vi "Test Person Broadcasts Status on Start.vi"(8 "error in (no error)":errorcluster, 11 "Person Test In":refnum<class "Person Test.lvclass">) -> (0 "error out":errorcluster, 3 "Person Test Out":refnum<class "Person Test.lvclass">)   [LabVIEW 2020, in "Person Test.lvclass"]
uses:
  Person Test/Person Test.lvclass
  C:/Program Files (x86)/National Instruments/LabVIEW 2020/vi.lib/Asteme/LUnit/Test Case.lvclass
  Processes/People/Person/Person.lvclass
  C:/Program Files (x86)/National Instruments/LabVIEW 2020/vi.lib/Asteme/Triarc Framework/Process/Process.lvclass
  <vilib>/Asteme/Triarc Framework/Process/Process.lvclass/Process.ctl
  <vilib>/Asteme/LUnit/Test Case.lvclass/Test Case.ctl
  <vilib>/Asteme/LUnit/LUnit Assertion Result.lvclass/LUnit Assertion Result.ctl
  <vilib>/Asteme/Triarc Framework Test Suite/Support/Execution timer.vi
  <vilib>/Asteme/Triarc Framework/Process/Private/SubVIs/Wait for finish.vi
  <vilib>/Asteme/Triarc Framework/Process/Protected/Messaging/Enqueue Message.vi
  <vilib>/Asteme/Triarc Framework/Process/Private/SubVIs/Set Lifecycle State.vi
  <vilib>/Asteme/Triarc Framework/Process/Public/Lifecycle/Get Lifecycle State.vi
  <vilib>/Asteme/LUnit/Palette/Fail.vi
  <vilib>/Asteme/LUnit/Palette/Pass.vi
  <vilib>/Asteme/LUnit/Variant to string.vi
  <vilib>/Asteme/LUnit/Set Assertion Type.vi
  <vilib>/Asteme/LUnit/Add test result.vi
  <vilib>/Asteme/LUnit/LUnit Get Test Case.vi
  <vilib>/Asteme/LUnit/Assertion Result/LUnit Get Test Name.vi
  <vilib>/Asteme/LUnit/LUnit Write Message.vi
  <vilib>/Asteme/LUnit/LUnit Write Description.vi
  <vilib>/Asteme/LUnit/LUnit Write Skipped.vi
  <vilib>/AdvancedString/1D String Array to Delimited String.vi
  <vilib>/Utility/error.llb/Clear Errors.vi
  <vilib>/Asteme/LUnit/LUnit Write Passed.vi
  <vilib>/Asteme/LUnit/LUnit Write Assertion Type.vi
  <vilib>/Asteme/LUnit/Read Test Case Name.vi
  <vilib>/Asteme/Triarc Framework Test Suite/Support/Event Helpers/Dequeue Event Message.vi
  <vilib>/Utility/error.llb/Error Cluster From Error Code.vi
  <vilib>/Utility/Data Type/Get Type Information.vi
  <vilib>/Utility/LVClass/Get LV Class Name.vi
  <vilib>/Asteme/LUnit/LUnit Assertion Result.lvclass
  <vilib>/Asteme/Triarc Framework/Process/Process.lvclass
  <vilib>/Asteme/Triarc Framework Test Suite/Support/Event Helpers/Event Helpers.lvlib
  <vilib>/Asteme/LUnit/Test Case.lvclass
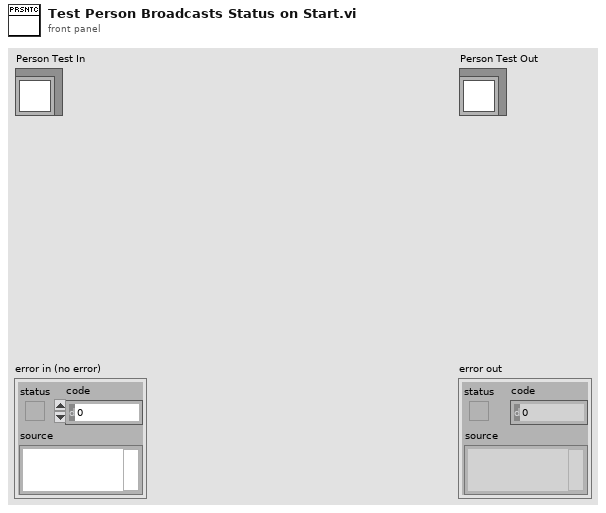
[diagram p1: front panel]
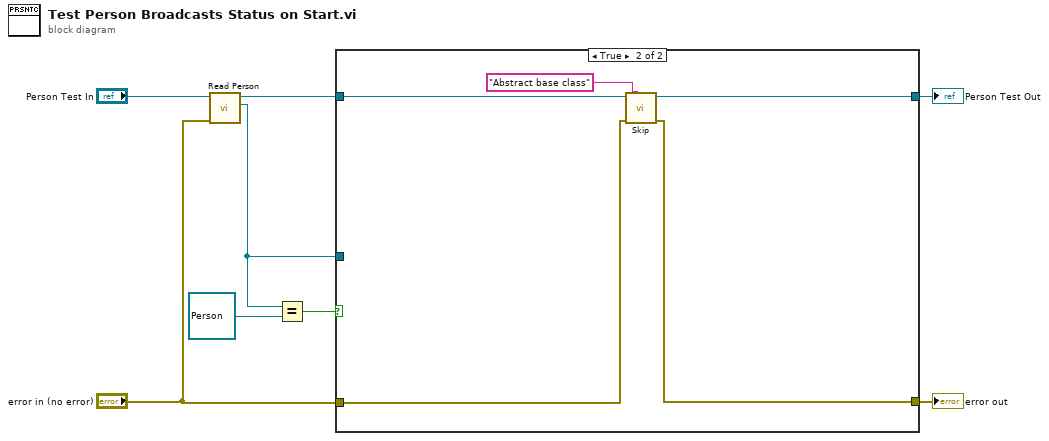
[diagram p0: block diagram]
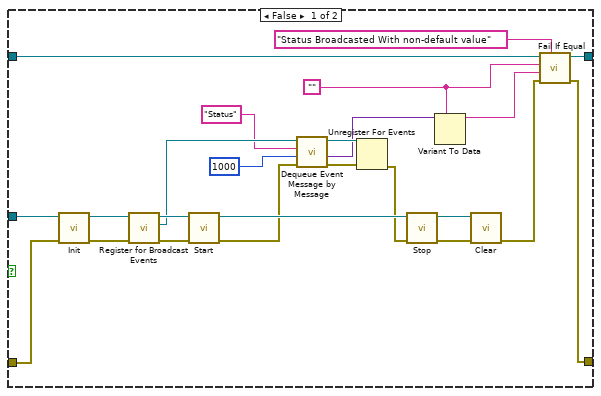
[diagram p2: hidden frame]
diagram:
  n1 = call "Read Person.vi"("error in (no error)"="error in (no error)", "Person Test in"="Person Test In") -> ("Person.lvclass"=w3:refnum<class "Person.lvclass">, "Person Test out"=w5:refnum<class "Person Test.lvclass">)  [unwired: 7 in, 1 out]
  n2 = Equal?(x=w3, y=refnum<class "Person.lvclass"> refnum ("Person.lvclass")) -> (x = y?=w1:bool)
  n3 = case shown="True" w1 {
    tunnel: [w22 w36] -> w8
    tunnel: [w18 w35] -> w7
    tunnel: w5 -> [w13 w37]
    tunnel: "error in (no error)" -> [w12 w34]
    tunnel: w3 -> [w9 _]
    frame False {
      w11 = ""
      n4 = call-dynamic "Init.vi"("error in (no error)"=w12, "View In"=w9) -> ("error out"=w29:errorcluster, "View Out"=w30:refnum<class "Person.lvclass">)  [unwired: 8 in]
      n5 = call <vilib>:"Register for Broadcast Events.vi"("error in (no error)"=w29, "Process In"=w30) -> ("error out"=w32:errorcluster, "Event Registration Refnum Out"=w26:refnum<event-registration>, "Process Out"=w31:refnum<class "Person.lvclass">)  [unwired: 7 in]
      n6 = call <vilib>:"Start.vi"("error in (no error)"=w32, "Process In"=w31) -> ("error out"=w24:errorcluster, "Process Out"=w25:refnum<class "Person.lvclass">)  [unwired: 8 in]
      n7 = call <vilib>:"Dequeue Event Message by Message.vi"("error in (no error)"=w24, "Timeout (-1)"=1000, "Message"="Status", "Event Registration Refnum"=w26) -> ("error out"=w23:errorcluster, "Message Data"=w14:variant, "Event Registration Refnum Out"=w17:refnum<event-registration>)  [unwired: 3 in, 2 out]
      n8 = Unregister For Events(event registration refnum=w17, error in=w23) -> (error out=w20:errorcluster)
      n9 = call <vilib>:"Stop.vi"("error in (no error)"=w20, "Process In"=w25) -> ("error out"=w27:errorcluster, "Process Out"=w28:refnum<class "Person.lvclass">)  [unwired: 7 in, 1 out]
      n10 = Variant To Data(type=w11, Variant=w14) -> (data=w10:string)  [unwired: 1 in, 1 out]
      n11 = call-dynamic "Clear.vi"("error in (no error)"=w27, "View In"=w28) -> ("error out"=w19:errorcluster)  [unwired: 9 in]
      n12 = call <vilib>:"Fail If Equal.vi"("Description"="Status Broadcasted With non-default value", "error in (no error)"=w19, "Actual"=w10, "Expected"=w11, "Test Case In"=w13) -> ("error out"=w18:errorcluster, "Test Case Out"=w22:refnum<class "Person Test.lvclass">)  [unwired: 5 in]
    }
    frame True {
      n13 = call <vilib>:"Skip.vi"("Description"="Abstract base class", "error in (no error)"=w34, "Test Case In"=w37) -> ("error out"=w35:errorcluster, "Test Case Out"=w36:refnum<class "Person Test.lvclass">)  [unwired: 7 in]
    }
  }
  "error out" <- w7
  "Person Test Out" <- w8
